vi "OP500_ZP_CMUSCAN.vi"(0 "Enable":bool=TRUE caption="Activer", 5 "error in (no error)":errorcluster caption="entrée d'erreur (pas d'erreur)") -> (15 "Température usine":dbl format="%#g", 16 "Nombre de températures":dbl format="%#g", 17 "Nombre de tensions":dbl format="%#g", 18 "OK":bool, 19 "error out":errorcluster caption="sortie d'erreur")   [LabVIEW 2020]
doc: "Affiche une boîte de dialogue standard qui invite l'utilisateur à entrer des informations, telles qu'un nom d'utilisateur et un mot de passe.\n--------------------\n\nCe VI Express est configuré comme suit :\n\nMessage à afficher à l'utilisateur :Renseigner les informations suivantes :\nLes entrées sont : \nNombre : Nombre de tensions\nNombre : Nombre de températures\nNombre : Température usine"
panel:
  in  "Température usine":dbl format="%#g"
  in  "Nombre de températures":dbl format="%#g"
  in  "Nombre de tensions":dbl format="%#g"
  out "String":string="Renseigner les informations suivantes :" caption="Chaîne"
  in  "Cancel":bool caption="Annuler"
  in  "OK2":bool
  in  "OK1":bool
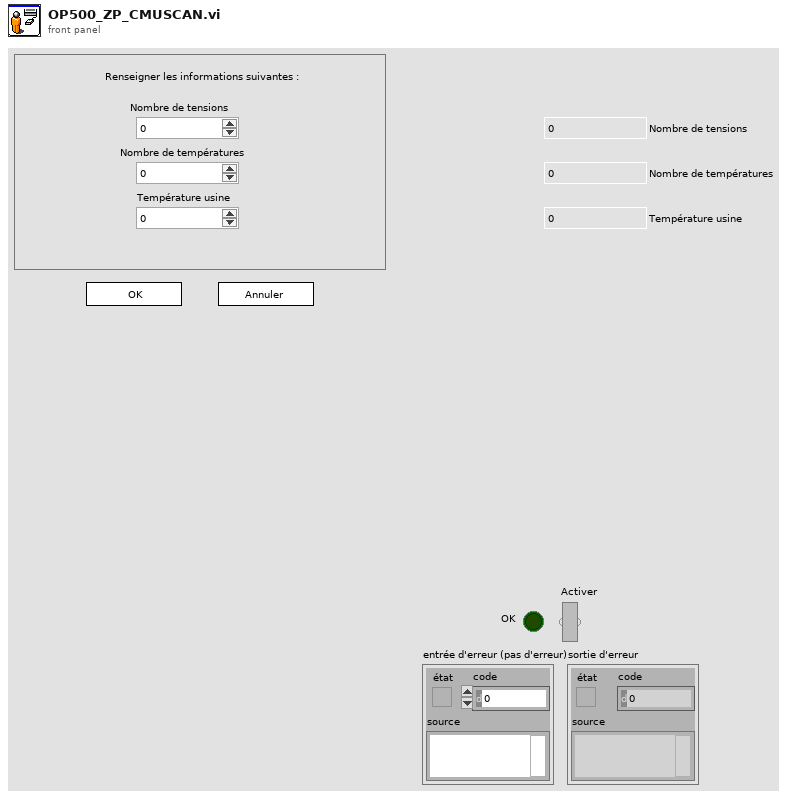
[diagram p1: front panel]
types:
  T1 = cluster{"Input Name":string, "Input Data Type":i32}[]
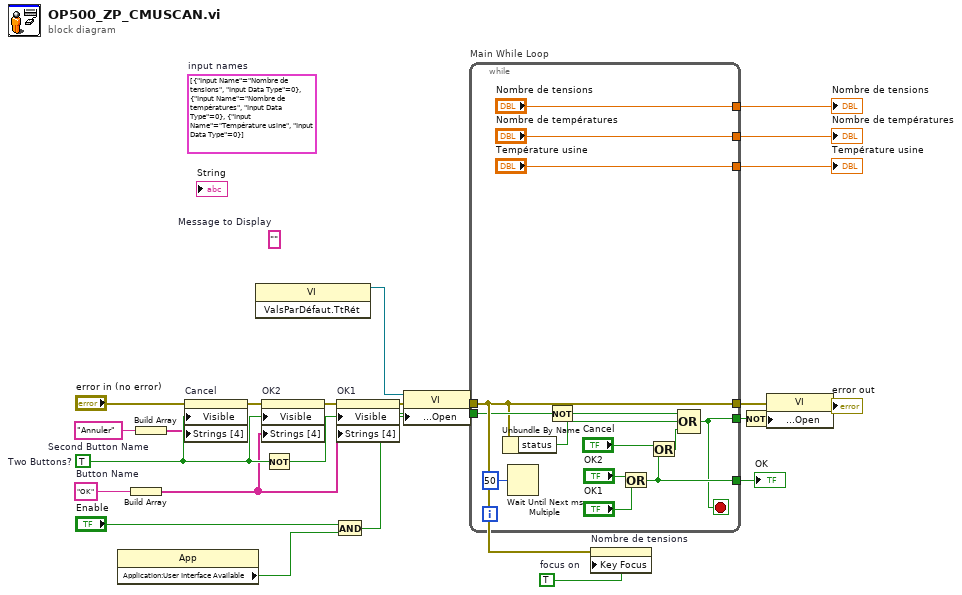
[diagram p0: block diagram]
diagram:
  w3 = TRUE  # focus on
  (unwired) T1 [{"Input Name"="Nombre de tensions", "Input Data Type"=0}, {"Input Name"="Nombre de températures", "Input Data Type"=0}, {"Input Name"="Température usine", "Input Data Type"=0}]  # input names
  w16 = "Annuler"  # Second Button Name
  w14 = "OK"  # Button Name
  (unwired) ""  # Message to Display
  w24 = TRUE  # Two Buttons?
  n1 = property class="App"() -> ("Application:User Interface Available"=w6:bool)  [unwired: 2 in, 2 out]
  n2 = Build Array(w14) -> (w15:string[])
  n3 = Build Array(w16) -> (w17:string[])
  n4 = property on="Cancel" class="Bool"(error in="error in (no error)", "Visible"=w24, "Strings [4]"=w17) -> (error out=w21:errorcluster)  [unwired: 1 in, 1 out]
  n5 = invoke class="VI" method="ValsParDéfaut.TtRét"() -> (reference out=w5:refnum<vi>)  [unwired: 3 in, 2 out]
  n6 = property on="OK2" class="Bool"(error in=w21, "Visible"=w24, "Strings [4]"=w15) -> (error out=w20:errorcluster)  [unwired: 1 in, 1 out]
  n7 = Not(x=w24) -> (.not. x?=w22:bool)
  n8 = And(x="Enable", y=w6) -> (x .and. y?=w7:bool)
  n9 = property on="OK1" class="Bool"(error in=w20, "Visible"=w22, "Strings [4]"=w15) -> (error out=w13:errorcluster)  [unwired: 1 in, 1 out]
  n10 = property class="VI"(reference=w5, error in=w13, "Front Panel Window:Open"=w7) -> (error out=w12:errorcluster)  [unwired: 1 out]
  n11 = while "Main While Loop" {
    tunnel: [w35] -> w23
    tunnel: w7 -> [w33]
    tunnel: [w31] -> w18
    tunnel: w12 -> [w30]
    tunnel: [w30] -> w10
    tunnel: ["Nombre de tensions"] -> w4
    tunnel: ["Nombre de températures"] -> w2
    tunnel: ["Température usine"] -> w1
    stop <- w31 stop-if-true
    n12 = Unbundle By Name(w30) -> ("status"=w28:bool)
    n13 = Wait Until Next ms Multiple(millisecond multiple=u32 50) -> ()  [unwired: 1 out]
    n14 = Not(x=w33) -> (.not. x?=w32:bool)
    n15 = Or(x="OK2", y="OK1") -> (x .or. y?=w35:bool)
    n16 = Or(x="Cancel", y=w35) -> (x .or. y?=w29:bool)
    n17 = Compound Arithmetic op=OR(w32, w28, w29) -> (w31:bool)
  }
  "OK" <- w23
  "Nombre de tensions" <- w4
  "Nombre de températures" <- w2
  "Température usine" <- w1
  n18 = property on="Nombre de tensions" class="NumNb (strict)"(error in=w12, "Key Focus"=w3) -> ()  [unwired: 1 in, 2 out]
  n19 = Not(x=w18) -> (.not. x?=w19:bool)
  n20 = property class="VI"(error in=w10, "Front Panel Window:Open"=w19) -> (error out=→"error out":errorcluster)  [unwired: 1 in, 1 out]
